vi "error.FormatErrorMessage.vi"(8 "error in (no error)":errorcluster) -> (1 "tag":T1, 2 "description":string, 3 "source":string)   [LabVIEW 2020]
uses:
  <vilib>/Utility/error.llb/TagReturnType.ctl
  <vilib>/Utility/error.llb/whitespace.ctl
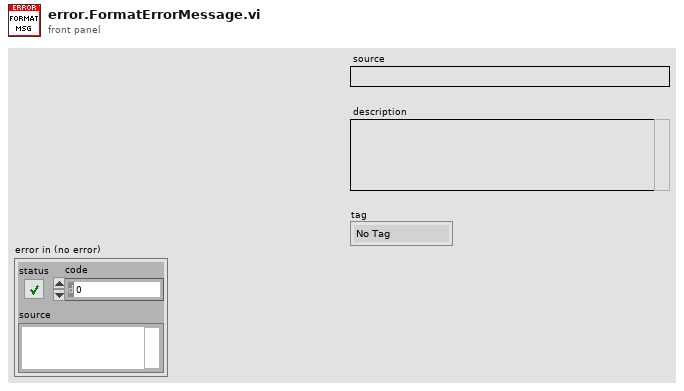
[diagram p1: front panel]
types:
  T1 = typedef "TagReturnType.ctl" = enum16{"No Tag", "<err>", "<append>"}
  T2 = typedef "whitespace.ctl" = u16
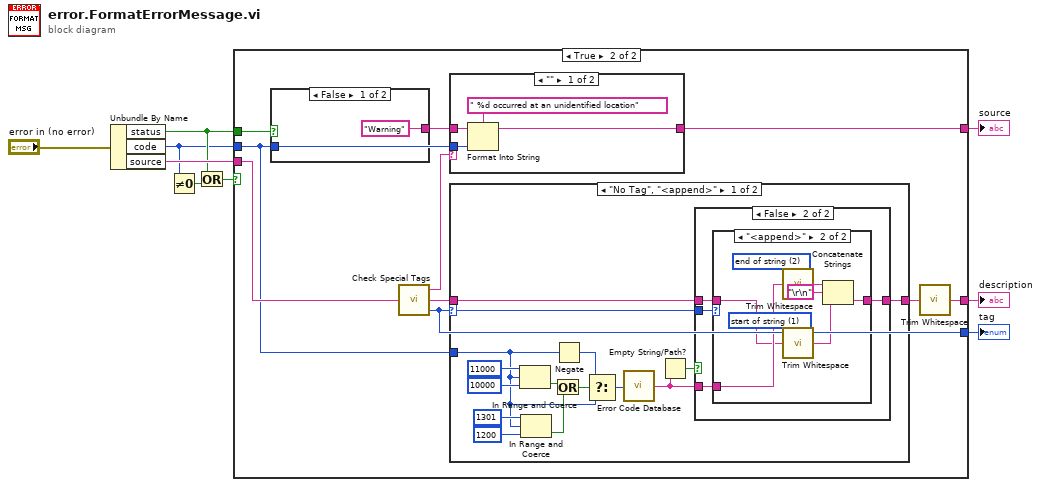
[diagram p0: block diagram]
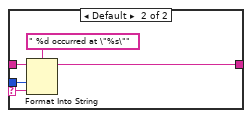
[diagram p3: hidden frame]
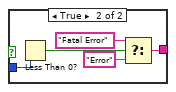
[diagram p4: hidden frame]
diagram:
  n1 = Unbundle By Name("error in (no error)") -> ("status"=w4:bool, "code"=w2:i32, "source"=w6:string)
  n2 = Not Equal To 0?(x=w2) -> (x != 0?=w3:bool)
  n3 = Or(x=w4, y=w3) -> (x .or. y?=w5:bool)
  n4 = case shown="True" w5 {
    tunnel: [_ w10] -> w9
    tunnel: [_ w18] -> w8
    tunnel: w2 -> [_ w12]
    tunnel: w6 -> [_ w16]
    tunnel: w4 -> [_ w15]
    tunnel: [_ w14] -> w1
    frame False {
    }
    frame True {
      n5 = case shown="False" w15 {
        tunnel: ["Warning" ("format string") w34] -> w13
        tunnel: w12 -> [_ w31]
        frame False {
        }
        frame True {
          n6 = Less Than 0?(x=w31) -> (x < 0?=w32:bool)
          n7 = Select(t="Fatal Error" ("format string"), s=w32, f="Error") -> (s? t:f=w34:string)
        }
      }
      n8 = call <vilib>:"Check Special Tags.vi"("source"=w16) -> ("Before Tag (source)"=w11:string, "After Tag (special data)"=w19:string, "Tag Found?"=w14:T1)
      n9 = case shown="\"\"" w11 {
        selector: w11 -> [_ w24]
        tunnel: [w23 w28] -> w10
        tunnel: w13 -> [w22 w27]
        tunnel: w12 -> [w21 w26]
        frame "" {
          n10 = Format Into String(format string=" %d occurred at an unidentified location", initial string=w22, w21) -> (resulting string=w23:string)  [unwired: 1 in, 1 out]
        }
        frame Default {
          n11 = Format Into String(format string=" %d occurred at \"%s\"", initial string=w27, w26, w24) -> (resulting string=w28:string)  [unwired: 1 in, 1 out]
        }
      }
      n12 = case shown="\"No Tag\", \"<append>\"" w14 {
        selector: w14 -> [w41 _]
        tunnel: [w39 w67] -> w17
        tunnel: w12 -> [w35 _]
        tunnel: w19 -> [w40 w67]
        frame "No Tag", "<append>" {
          n13 = In Range and Coerce(upper limit=11000, x=w35, lower limit=10000) -> (In Range?=w44:bool)  [unwired: 1 out]
          n14 = In Range and Coerce(upper limit=1301, x=w35, lower limit=1200) -> (In Range?=w45:bool)  [unwired: 1 out]
          n15 = Or(x=w44, y=w45) -> (x .or. y?=w43:bool)
          n16 = Negate(x=w35) -> (-x=w47:i32)
          n17 = Select(t=w47, s=w43, f=w35) -> (s? t:f=w38:i32)
          n18 = call <vilib>:"Error Code Database.vi"("Error Code"=w38) -> ("Error Text"=w37:string)
          n19 = Empty String/Path?(string/path=w37) -> (empty?=w36:bool)
          n20 = case shown="False" w36 {
            tunnel: [w52 w55] -> w39
            tunnel: w37 -> [_ w54]
            tunnel: w41 -> [w50 w57]
            tunnel: w40 -> [w51 w56]
            frame True {
              n21 = case shown="\"<append>\"" w50 {
                tunnel: [_ w53] -> w52
                tunnel: w51 -> [_ w53]
                frame "No Tag", Default {
                  # "Code is undefined..."
                }
                frame "<append>" {
                }
              }
            }
            frame False {
              n22 = case shown="\"<append>\"" w57 {
                tunnel: w54 -> [w58 w62]
                tunnel: [w58 w65] -> w55
                tunnel: w56 -> [_ w61]
                frame "No Tag", Default {
                }
                frame "<append>" {
                  w59 = T2 1 items=["both", "start of string", "end of string"] ("location (both)")
                  w64 = T2 2 items=["both", "start of string", "end of string"] ("location (both)")
                  n23 = call <vilib>:"Trim Whitespace.vi"("string"=w62, "location (both)"=w64) -> ("trimmed string"=w63:string)
                  n24 = call <vilib>:"Trim Whitespace.vi"("string"=w61, "location (both)"=w59) -> ("trimmed string"=w60:string)
                  n25 = Concatenate Strings(w63, "\r\n" ("End of Line Constant"), w60) -> (w65:string)
                }
              }
            }
          }
        }
        frame "<err>" {
        }
      }
      n26 = call <vilib>:"Trim Whitespace.vi"("string"=w17) -> ("trimmed string"=w18:string)  [unwired: 1 in]
    }
  }
  "source" <- w9
  "description" <- w8
  "tag" <- w1
